vi "TrackColorM.vi"() -> ()   [LabVIEW 2015]
panel:
  out "Bounding Box[0].x":sgl
  in  "Line Coordinates":i32[](array[numeric])
  in  "Stop (F)":bool
  out "Image Out":T1(plugin-control)
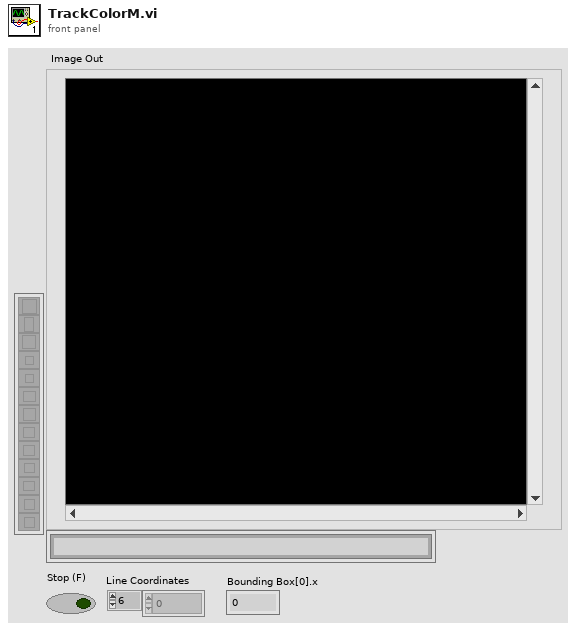
[diagram p1: front panel]
types:
  T1 = typedef "IMAQ Image.ctl" = refnum<image>
  T2 = typedef "Image Type" = u32
  T3 = cluster{"Position":cluster{"x":sgl, "y":sgl}, "Angle":sgl, "Scale":sgl, "Score":sgl, "Bounding Box":cluster{"x":sgl, "y":sgl}[]}[]
  T4 = cluster{"Matches (Color Location 1)[0]":cluster{"Position":cluster{"x":sgl, "y":sgl}, "Angle":sgl, "Scale":sgl, "Score":sgl, "Bounding Box":cluster{"x":sgl, "y":sgl}[]}, "Matches (Color Location 1)[1]":cluster{"Position":cluster{"x":sgl, "y":sgl}, "Angle":sgl, "Scale":sgl, "Score":sgl, "Bounding Box":cluster{"x":sgl, "y":sgl}[]}, "Matches (Color Location 1)[2]":cluster{"Position":cluster{"x":sgl, "y":sgl}, "Angle":sgl, "Scale":sgl, "Score":sgl, "Bounding Box":cluster{"x":sgl, "y":sgl}[]}, "Matches (Color Location 1)[3]":cluster{"Position":cluster{"x":sgl, "y":sgl}, "Angle":sgl, "Scale":sgl, "Score":sgl, "Bounding Box":cluster{"x":sgl, "y":sgl}[]}}
  T5 = cluster{"Matches (Color Location 2)[0]":cluster{"Position":cluster{"x":sgl, "y":sgl}, "Angle":sgl, "Scale":sgl, "Score":sgl, "Bounding Box":cluster{"x":sgl, "y":sgl}[]}, "Matches (Color Location 2)[1]":cluster{"Position":cluster{"x":sgl, "y":sgl}, "Angle":sgl, "Scale":sgl, "Score":sgl, "Bounding Box":cluster{"x":sgl, "y":sgl}[]}, "Matches (Color Location 2)[2]":cluster{"Position":cluster{"x":sgl, "y":sgl}, "Angle":sgl, "Scale":sgl, "Score":sgl, "Bounding Box":cluster{"x":sgl, "y":sgl}[]}, "Matches (Color Location 2)[3]":cluster{"Position":cluster{"x":sgl, "y":sgl}, "Angle":sgl, "Scale":sgl, "Score":sgl, "Bounding Box":cluster{"x":sgl, "y":sgl}[]}}
  T6 = cluster{"Matches (Color Location 3)[0]":cluster{"Position":cluster{"x":sgl, "y":sgl}, "Angle":sgl, "Scale":sgl, "Score":sgl, "Bounding Box":cluster{"x":sgl, "y":sgl}[]}, "Matches (Color Location 3)[1]":cluster{"Position":cluster{"x":sgl, "y":sgl}, "Angle":sgl, "Scale":sgl, "Score":sgl, "Bounding Box":cluster{"x":sgl, "y":sgl}[]}, "Matches (Color Location 3)[2]":cluster{"Position":cluster{"x":sgl, "y":sgl}, "Angle":sgl, "Scale":sgl, "Score":sgl, "Bounding Box":cluster{"x":sgl, "y":sgl}[]}, "Matches (Color Location 3)[3]":cluster{"Position":cluster{"x":sgl, "y":sgl}, "Angle":sgl, "Scale":sgl, "Score":sgl, "Bounding Box":cluster{"x":sgl, "y":sgl}[]}}
  T7 = cluster{"Bounding Box[0]":cluster{"x":sgl, "y":sgl}, "Bounding Box[1]":cluster{"x":sgl, "y":sgl}, "Bounding Box[2]":cluster{"x":sgl, "y":sgl}, "Bounding Box[3]":cluster{"x":sgl, "y":sgl}}
  T8 = cluster{"[0]":sgl, "[1]":sgl, "[2]":sgl, "[3]":sgl}
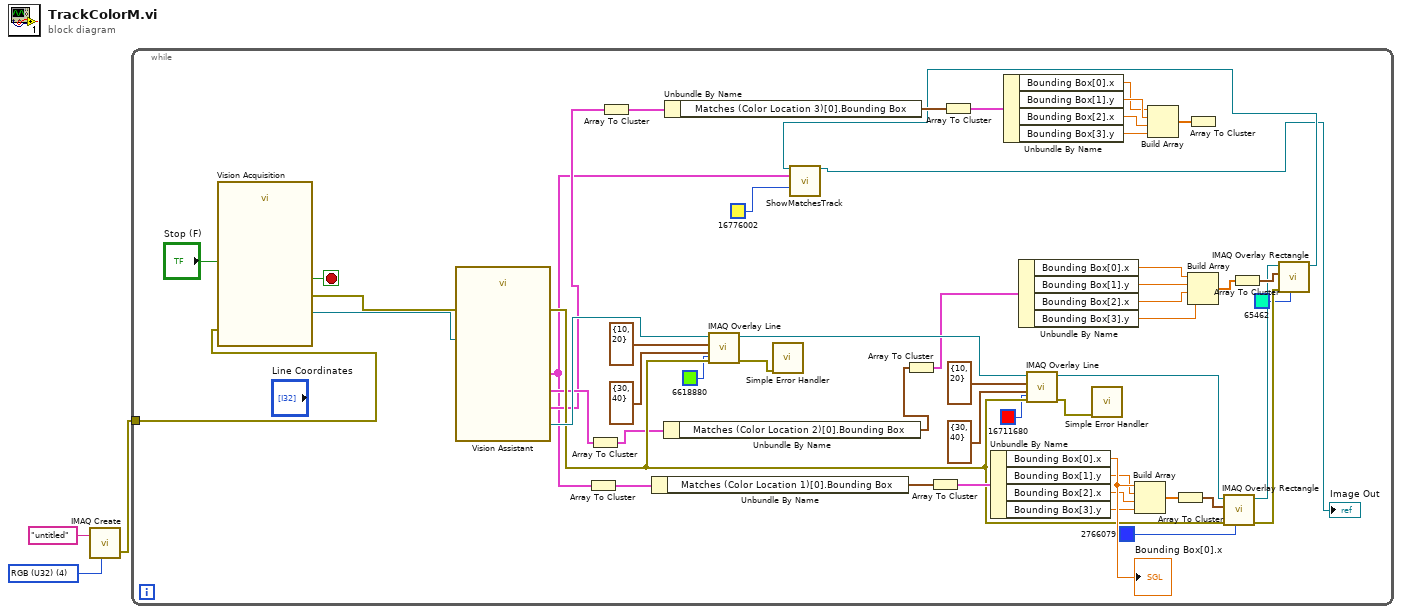
[diagram p0: block diagram]
diagram:
  w2 = T2 4 items=["Grayscale (U8)", "Grayscale (I16)", "Grayscale (SGL)", "Complex (CSG)", "RGB (U32)", "HSL (U32)", "RGB (U64)", "Grayscale (U16)"] ("Image Type")
  n1 = call "IMAQ Create"("Image Name"="untitled", "Image Type"=w2) -> ("error out"=w1:errorcluster)  [unwired: 3 in, 1 out]
  n2 = while {
    tunnel: w1 -> [w33]
    stop <- w55 stop-if-true
    n3 = call "Vision Acquisition"("Stop (F)"="Stop (F)", "error in"=w33) -> ("Image Out"=w34:T1, "Stopped"=w55:bool, "error out"=w32:errorcluster)  [unwired: 23 in]
    n4 = call "Vision Assistant"("Image In"=w34, "error in"=w32) -> ("Image Out"=w44:T1, "Matches (Color Location 1)"=w4:T3, "Matches (Color Location 2)"=w29:T3, "Matches (Color Location 3)"=w8:T3, "error out"=w43:errorcluster)  [unwired: 21 in]
    n5 = Array To Cluster(array=w4) -> (cluster=w31:T4)
    n6 = Array To Cluster(array=w29) -> (cluster=w30:T5)
    n7 = Array To Cluster(array=w8) -> (cluster=w10:T6)
    n8 = Unbundle By Name(w31) -> ("Matches (Color Location 1)[0].Bounding Box"=w54:cluster{"x":sgl, "y":sgl}[])
    n9 = Unbundle By Name(w30) -> ("Matches (Color Location 2)[0].Bounding Box"=w28:cluster{"x":sgl, "y":sgl}[])
    n10 = Unbundle By Name(w10) -> ("Matches (Color Location 3)[0].Bounding Box"=w16:cluster{"x":sgl, "y":sgl}[])
    n11 = call "IMAQ Overlay Line"("Color"=u32 6618880, "error in (no error)"=w43, "End Point"=cluster{"X":i32, "Y":i32} {"X"=30, "Y"=40} ("Start Point"), "Start Point"=cluster{"X":i32, "Y":i32} {"X"=10, "Y"=20}, "Image"=w44) -> ("error out"=w36:errorcluster, "Image Out"=w45:T1)  [unwired: 5 in]
    n12 = call <vilib>:"Simple Error Handler.vi"("error in (no error)"=w36) -> ()  [unwired: 4 in, 5 out]
    n13 = Array To Cluster(array=w28) -> (cluster=w27:T7)
    n14 = Array To Cluster(array=w54) -> (cluster=w53:T7)
    n15 = Array To Cluster(array=w16) -> (cluster=w15:T7)
    n16 = Unbundle By Name(w53) -> ("Bounding Box[0].x"=w52:sgl, "Bounding Box[1].y"=w49:sgl, "Bounding Box[2].x"=w50:sgl, "Bounding Box[3].y"=w51:sgl)
    "Bounding Box[0].x" <- w52
    n17 = Unbundle By Name(w15) -> ("Bounding Box[0].x"=w9:sgl, "Bounding Box[1].y"=w12:sgl, "Bounding Box[2].x"=w13:sgl, "Bounding Box[3].y"=w14:sgl)
    n18 = Unbundle By Name(w27) -> ("Bounding Box[0].x"=w26:sgl, "Bounding Box[1].y"=w25:sgl, "Bounding Box[2].x"=w24:sgl, "Bounding Box[3].y"=w23:sgl)
    n19 = call "IMAQ Overlay Line"("Color"=u32 16711680, "error in (no error)"=w43, "End Point"=cluster{"X":i32, "Y":i32} {"X"=30, "Y"=40} ("Start Point"), "Start Point"=cluster{"X":i32, "Y":i32} {"X"=10, "Y"=20}, "Image"=w45) -> ("error out"=w35:errorcluster, "Image Out"=w46:T1)  [unwired: 5 in]
    n20 = call <vilib>:"Simple Error Handler.vi"("error in (no error)"=w35) -> ()  [unwired: 4 in, 5 out]
    n21 = Build Array(w52, w49, w50, w51) -> (w48:sgl[])
    n22 = Build Array(w9, w12, w13, w14) -> (w11:sgl[])
    n23 = Array To Cluster(array=w48) -> (cluster=w47:T8)
    n24 = Array To Cluster(array=w11) -> ()  [unwired: 1 out]
    n25 = Build Array(w26, w25, w24, w23) -> (w22:sgl[])
    n26 = call "IMAQ Overlay Rectangle"("Color"=u32 2766079, "error in (no error)"=w43, "Rectangle"=w47, "Image"=w46) -> ("error out"=w19:errorcluster, "Image Out"=w20:T1)  [unwired: 6 in]
    n27 = Array To Cluster(array=w22) -> (cluster=w21:T8)
    n28 = call "IMAQ Overlay Rectangle"("Color"=u32 65462, "error in (no error)"=w19, "Rectangle"=w21, "Image"=w20) -> ("Image Out"=w7:T1)  [unwired: 6 in, 1 out]
    n29 = call "ShowMatchesTrack.vi"("Refnum in"=w7, "Matches (Color Location 3)"=w4, "Color"=u32 16776002) -> ("Refnum out"=→"Image Out":T1)  [unwired: 8 in, 4 out]
  }
